vi "List Program.vi"(4 "error in (no error)":errorcluster, 6 "Program Number (1)":i32=1 min=1 max=100, 7 "VISA resource name":refnum<visa-resource-name>) -> (0 "error out":errorcluster, 2 "List Program":string, 3 "VISA resource name out":refnum<visa-resource-name>)   [LabVIEW 2015, in "Newport ESP301.lvlib"]
doc: "This command reads a specified program from non-volatile memory and sends it to the selected communication port (RS232 or IEEE488). During the transmission no other command should be sent to the controller.\nNote\nThe program list always terminates with the word “END”"
uses:
  Newport ESP301.lvlib
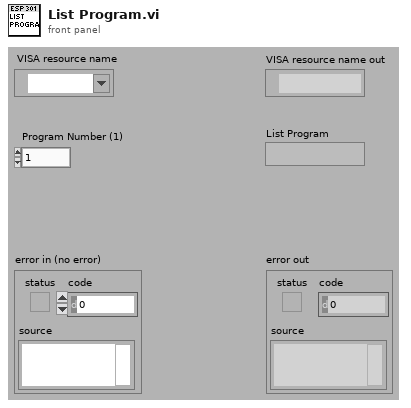
[diagram p1: front panel]
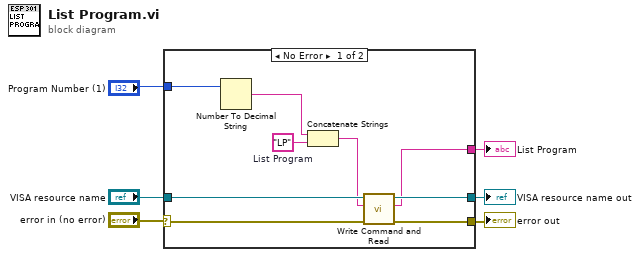
[diagram p0: block diagram]
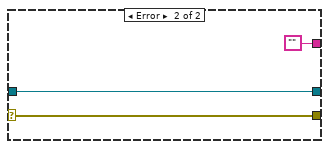
[diagram p2: hidden frame]
diagram:
  n1 = case shown="No Error" "error in (no error)" {
    selector: "error in (no error)" -> [w12 w18]
    tunnel: [w14 w18] -> w6
    tunnel: "VISA resource name" -> [w15 w17]
    tunnel: [w13 w17] -> w5
    tunnel: "Program Number (1)" -> [w8 _]
    tunnel: [w7 ""] -> w1
    frame No Error {
      w11 = "LP"  # List Program
      n2 = Number To Decimal String(number=w8) -> (decimal integer string=w10:string)  [unwired: 1 in]
      n3 = Concatenate Strings(w10, w11) -> (w9:string)
      n4 = call "Write Command and Read.vi"("error in (no error)"=w12, "Command"=w9, "VISA resource name"=w15) -> ("error out"=w14:errorcluster, "Returned string"=w7:string, "VISA resource name out"=w13:refnum<visa-resource-name>)  [unwired: 4 in]
    }
    frame Error {
    }
  }
  "error out" <- w6
  "VISA resource name out" <- w5
  "List Program" <- w1
